vi "EnableDisable - Right Click.vi"(0 "Node Ptr":T1 format="%.0x") -> ()   [LabVIEW 2024, in "Embedded TDMS Logger System Explorer.lvlib"]
doc: "Allows the user to enable or disable the custom device at any time. Is very useful during debugging sessions to be able to remove a custom device from operation without deleting it."
uses:
  Embedded TDMS Logger System Explorer.lvlib
  <vilib>/NI VeriStand/Custom Device API/Custom Device Item Ref.ctl
  Shared/Constants.vi
  <vilib>/NI VeriStand/Custom Device API/Custom Device API.lvlib
  Shared/Embedded TDMS Logger Shared.lvlib
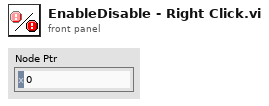
[diagram p1: front panel]
types:
  T1 = typedef "Custom Device API.lvlib/Custom Device Item Ref.ctl" = u64
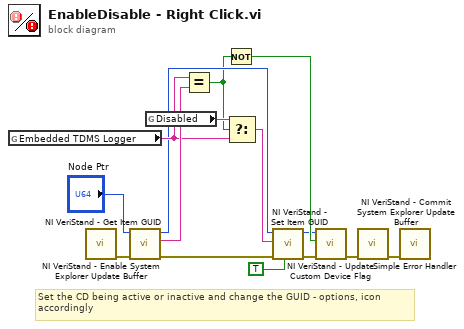
[diagram p0: block diagram]
diagram:
  # "Set the CD being active or inactive and change the GUID - options, icon\naccordingly"
  n1 = global read "Constants.vi" "Embedded TDMS Logger"() -> (w13:string)
  n2 = call <vilib>:"NI VeriStand - Enable System Explorer Update Buffer.vi"() -> ("error out"=w4:errorcluster)  [unwired: 11 in]
  n3 = call <vilib>:"NI VeriStand - Get Item GUID.vi"("error in (no error)"=w4, "Item Ref in"="Node Ptr") -> ("error out"=w9:errorcluster, "GUID"=w15:string, "Item Ref out"=w10:T1)  [unwired: 7 in]
  n4 = global read "Constants.vi" "Disabled"() -> (w12:string)
  n5 = Equal?(x=w13, y=w15) -> (x = y?=w8:bool)
  n6 = Not(x=w8) -> (.not. x?=w7:bool)
  n7 = Select(t=w12, s=w8, f=w13) -> (s? t:f=w11:string)
  n8 = call <vilib>:"NI VeriStand - Set Item GUID.vi"("Refresh System Explorer Tree? (F)"=TRUE, "error in (no error)"=w9, "GUID"=w11, "Item Ref in"=w10) -> ("error out"=w5:errorcluster, "Item Ref out"=w6:T1)  [unwired: 6 in]
  n9 = call <vilib>:"NI VeriStand - Update Custom Device Flag.vi"("error in (no error)"=w5, "Is Custom Device Active?"=w7, "Device Ref in"=w6) -> ("error out"=w3:errorcluster)  [unwired: 7 in, 1 out]
  n10 = call <vilib>:"NI VeriStand - Commit System Explorer Update Buffer.vi"("error in (no error)"=w3) -> ("error out"=w2:errorcluster)  [unwired: 10 in]
  n11 = call <vilib>:"Simple Error Handler.vi"("error in (no error)"=w2) -> ()  [unwired: 4 in, 5 out]
